vi "Set ToolStripProgressBar Width.vi"(8 "error in (no error)":errorcluster caption="错误输入（无错误）", 10 "Width":i32, 11 "ToolStripProgressBar 输入":refnum<class "ToolStripProgressBar.lvclass"> caption="DNL_LabVIEW Object in") -> (0 "error out":errorcluster caption="错误输出", 3 "ToolStripProgressBar 输出":refnum<class "ToolStripProgressBar.lvclass"> caption="DNL_LabVIEW Object out")   [LabVIEW 2013, in "ToolStripProgressBar.lvclass"]
uses:
  ToolStripProgressBar.lvclass
  ToolStripProgressBar.lvclass/ToolStripProgressBar.ctl
  System.Windows.Forms
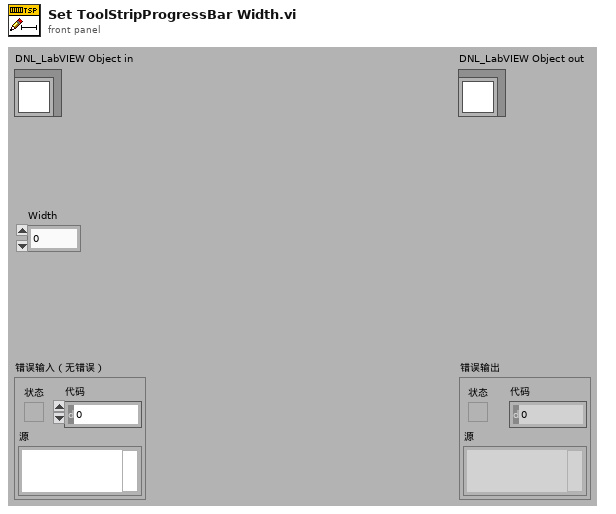
[diagram p1: front panel]
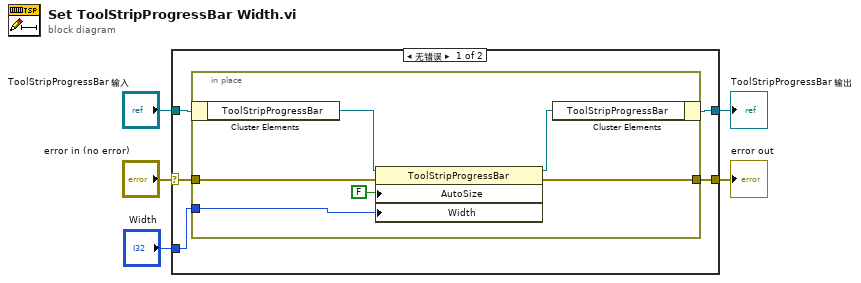
[diagram p0: block diagram]
diagram:
  n1 = case shown="无错误" "error in (no error)" {
    selector: "error in (no error)" -> [w8 w18]
    tunnel: [w7 w18] -> w4
    tunnel: [w6 w17] -> w2
    tunnel: "ToolStripProgressBar 输入" -> [w10 w17]
    tunnel: "Width" -> [w9 _]
    frame No Error {
      n2 = in-place {
        in-place-border: w9 -> [w11]
        in-place-border: w8 -> [w14]
        in-place-border: [w13] -> w7
        n3 = in-place-cluster #1(w10) -> ("ToolStripProgressBar"=w16:refnum<k24>)
        n4 = property class="ToolStripProgressBar"(reference=w16, error in=w14, "AutoSize"=FALSE, "Width"=w11) -> (reference out=w15:refnum<k24>, error out=w13:errorcluster)
        n5 = in-place-cluster #1("ToolStripProgressBar"=w15) -> (w6:refnum<class "ToolStripProgressBar.lvclass">)
      }
    }
    frame Error {
    }
  }
  "error out" <- w4
  "ToolStripProgressBar 输出" <- w2
